vi "HandleAcquisition.vi"(8 "error in (no error)":errorcluster, 10 "ID":u32, 11 "S4ACS_GUI in":refnum<class "S4ACS_GUI.lvclass">) -> (0 "error out":errorcluster, 3 "S4ACS_GUI out":refnum<class "S4ACS_GUI.lvclass">)   [LabVIEW 2018, in "S4ACS_GUI.lvclass"]
uses:
  S4ACS_GUI.lvclass
  S4ACS_GUI.lvclass/S4ACS_GUI.ctl
  Acquisition/Acquisition.lvclass
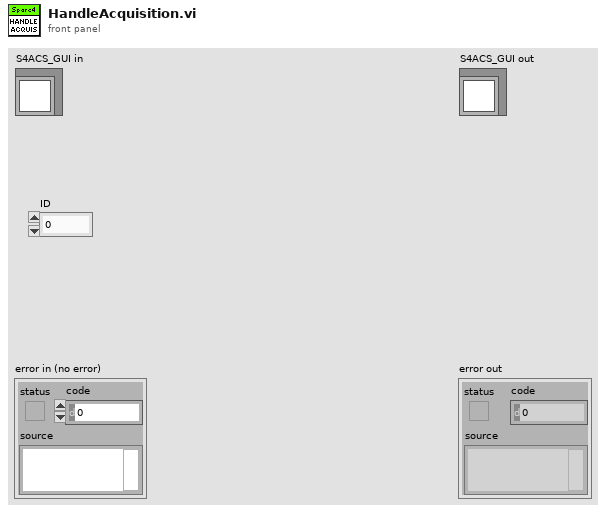
[diagram p1: front panel]
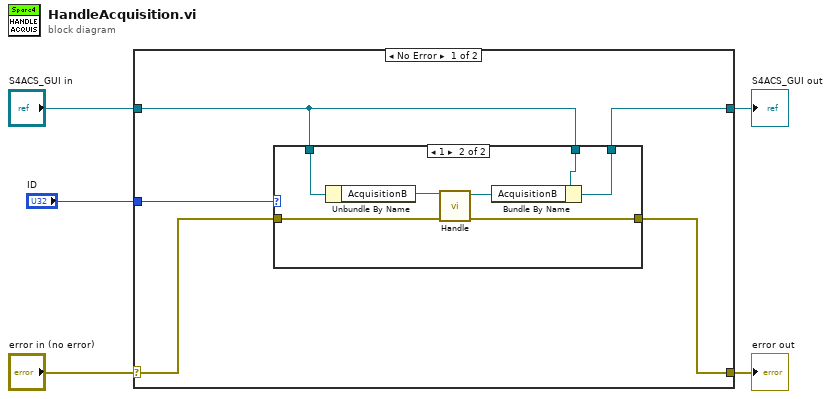
[diagram p0: block diagram]
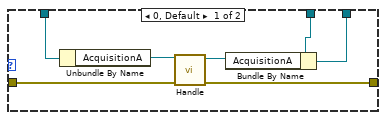
[diagram p2: hidden frame]
diagram:
  n1 = case shown="No Error" "error in (no error)" {
    selector: "error in (no error)" -> [w7 w26]
    tunnel: [w6 w26] -> w4
    tunnel: [w8 w25] -> w2
    tunnel: "S4ACS_GUI in" -> [w9 w25]
    tunnel: "ID" -> [w10 _]
    frame No Error {
      n2 = case shown="1" w10 {
        tunnel: w9 -> [w17 w24]
        tunnel: w9 -> [w15 w22]
        tunnel: [w14 w21] -> w8
        tunnel: w7 -> [w12 w19]
        tunnel: [w11 w18] -> w6
        frame 0, Default {
          n3 = Unbundle By Name(w17) -> ("AcquisitionA"=w16:refnum<class "Acquisition.lvclass">)
          n4 = call-dynamic "Handle.vi"("error in (no error)"=w12, "Acquisition in"=w16) -> ("error out"=w11:errorcluster, "Acquisition out"=w13:refnum<class "Acquisition.lvclass">)  [unwired: 8 in]
          n5 = Bundle By Name(cluster=w15, "AcquisitionA"=w13) -> (w14:refnum<class "S4ACS_GUI.lvclass">)
        }
        frame 1 {
          n6 = Unbundle By Name(w24) -> ("AcquisitionB"=w23:refnum<class "Acquisition.lvclass">)
          n7 = call-dynamic "Handle.vi"("error in (no error)"=w19, "Acquisition in"=w23) -> ("error out"=w18:errorcluster, "Acquisition out"=w20:refnum<class "Acquisition.lvclass">)  [unwired: 8 in]
          n8 = Bundle By Name(cluster=w22, "AcquisitionB"=w20) -> (w21:refnum<class "S4ACS_GUI.lvclass">)
        }
      }
    }
    frame Error {
    }
  }
  "error out" <- w4
  "S4ACS_GUI out" <- w2
